vi "Main.vi"(11 "Module Admin":refnum<class "Delacor_lib_QMH_Module Admin.lvclass">) -> ()   [LabVIEW 2024, in "Singleton.lvlib"]
doc: "This template is based off of the Queued Message Handler design pattern and the Queued Message Handler project template that ships with LabVIEW.\n\nThe main difference is that the queue is private to this module and communication between modules is performed via Broadcast and Request events.\n\nRequest events are wrapped in public API methods and are handled in the Event Handling Loop (EHL) of this VI. Any module can register for Broadcast events sent by this module. The EHL generates messages based on user interface actions.\n\nThe Message Handling Loop (MHL) processes messages generated by the EHL, or by other messages. The messages are string values, so new messages can be added easily to the Message Cases case structure in the MHL. Each message cluster can also provide an optional value for Message Data, which is a variant that can be converted to whatever message-specific data is required.\n_____\nBased on DQMH Dev Tools: Project Template 7.1.0.1464."
uses:
  Singleton.lvlib
  <vilib>/Delacor/Delacor QMH/Libraries/Module Admin_class/Delacor_lib_QMH_Module Admin.lvclass
  Module Data--cluster.ctl
  Do Something Argument--cluster.ctl
  <vilib>/Delacor/Delacor QMH/Libraries/Message Queue_class/Delacor_lib_QMH_Message Queue.lvclass/Delacor_lib_QMH_Message Queue.ctl
  Do Something Else Argument--cluster.ctl
  Do Something Else and Wait for Reply Argument--cluster.ctl
  Do Something Else and Wait (Reply Payload)--cluster.ctl
  Stop Argument--cluster.ctl
  <vilib>/Delacor/Delacor QMH/Libraries/Module Admin_class/Delacor_lib_QMH_Module Admin.lvclass/Delacor_lib_QMH_Module Admin.ctl
  New Event Argument--cluster.ctl
  <vilib>/Utility/miscctls.llb/LVPointTypeDef.ctl
  <vilib>/Delacor/Delacor QMH/Libraries/Message Queue_class/Delacor_lib_QMH_Enqueue Message (Single).vi
  <vilib>/Delacor/Delacor QMH/Libraries/Module Admin_class/Delacor_lib_QMH_Get External Launch.vi
  <vilib>/JKI/JKI Simple Localization/Private/RegisterVIJKI_Simple_Localization.vi
  <vilib>/Delacor/Delacor QMH/Libraries/Message Queue_class/Delacor_lib_QMH_Message Queue.lvclass
  <vilib>/JKI/JKI Simple Localization/API/JKI Simple LocalizationJKI_Simple_Localization.lvlib
panel:
  out "error out":errorcluster
  out "X":dbl
  out "Status":string
  in  "Simulate MHL Error":bool
  in  "Simulate EHL Error":bool
  in  "Do Something Else <Replace Me>":bool
  in  "Do Something <Replace Me>":bool
  # "These controls have associated \"Value Changed\" events configured in the Event Structure on the diagram.\n\nReplace them (and reconfigure the Event Structure) with the controls you need for your application. \n\nOther processes communicate with this Module via its Public API (wrappers for its Request Events).\n\nThis Module communicates with other processes via its Broadcast Events.\nAny process that wants to receive these messages can register for this module's Broadcast events."
  # "This template is for the DQMH framework. See the block diagram for more information on how to use this template."
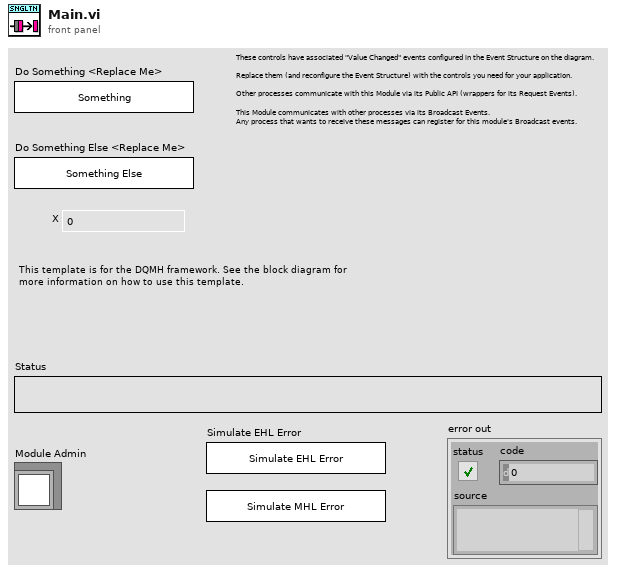
[diagram p1: front panel]
types:
  T1 = typedef "Singleton.lvlib/Request Events--cluster.ctl" = cluster{"Stop Module":refnum<user-event>, "Do Something":refnum<user-event>, "Do Something Else":refnum<user-event>, "Do Something Else and Wait for Reply":refnum<user-event>, "Show Panel":refnum<user-event>, "Hide Panel":refnum<user-event>, "Get Module Execution Status":refnum<user-event>, "Show Diagram":refnum<user-event>, "New Event":refnum<user-event>, "NEW EVENT TO HL":refnum<user-event>}
  T2 = typedef "Singleton.lvlib/Module Data--cluster.ctl" = cluster{"Status":string}
  T3 = typedef "Singleton.lvlib/Do Something Argument--cluster.ctl" = cluster{"Do Something Msg":string}
  T4 = typedef "Singleton.lvlib/Do Something Else Argument--cluster.ctl" = cluster{"Do Something Else Msg":string, "X":dbl}
  T5 = typedef "Singleton.lvlib/Do Something Else and Wait for Reply Argument--cluster.ctl" = cluster{"Do Something Else Msg":string, "X":dbl, "Wait Notifier":refnum<notifier>, "wait for reply":bool}
  T6 = enum32{"invalid lock state", "Not Locked", "Locked (No Password)", "Password-protected"}
  T7 = typedef "Singleton.lvlib/Stop Argument--cluster.ctl" = cluster{"Origin":string, "Exit via Stop Module Req?":bool, "Wait for Module to stop?":bool}
  T8 = typedef "Singleton.lvlib/New Event Argument--cluster.ctl" = cluster{"Numeric":dbl}
  T9 = typedef "LVPointTypeDef.ctl" = cluster{"Horizontal":i16, "Vertical":i16}
  T10 = enum32{"Invalid", "Standard", "Closed", "Hidden", "Minimized", "Maximized"}
  T11 = typedef "Singleton.lvlib/Do Something Else and Wait (Reply Payload)--cluster.ctl" = cluster{"Value":dbl, "error":errorcluster}
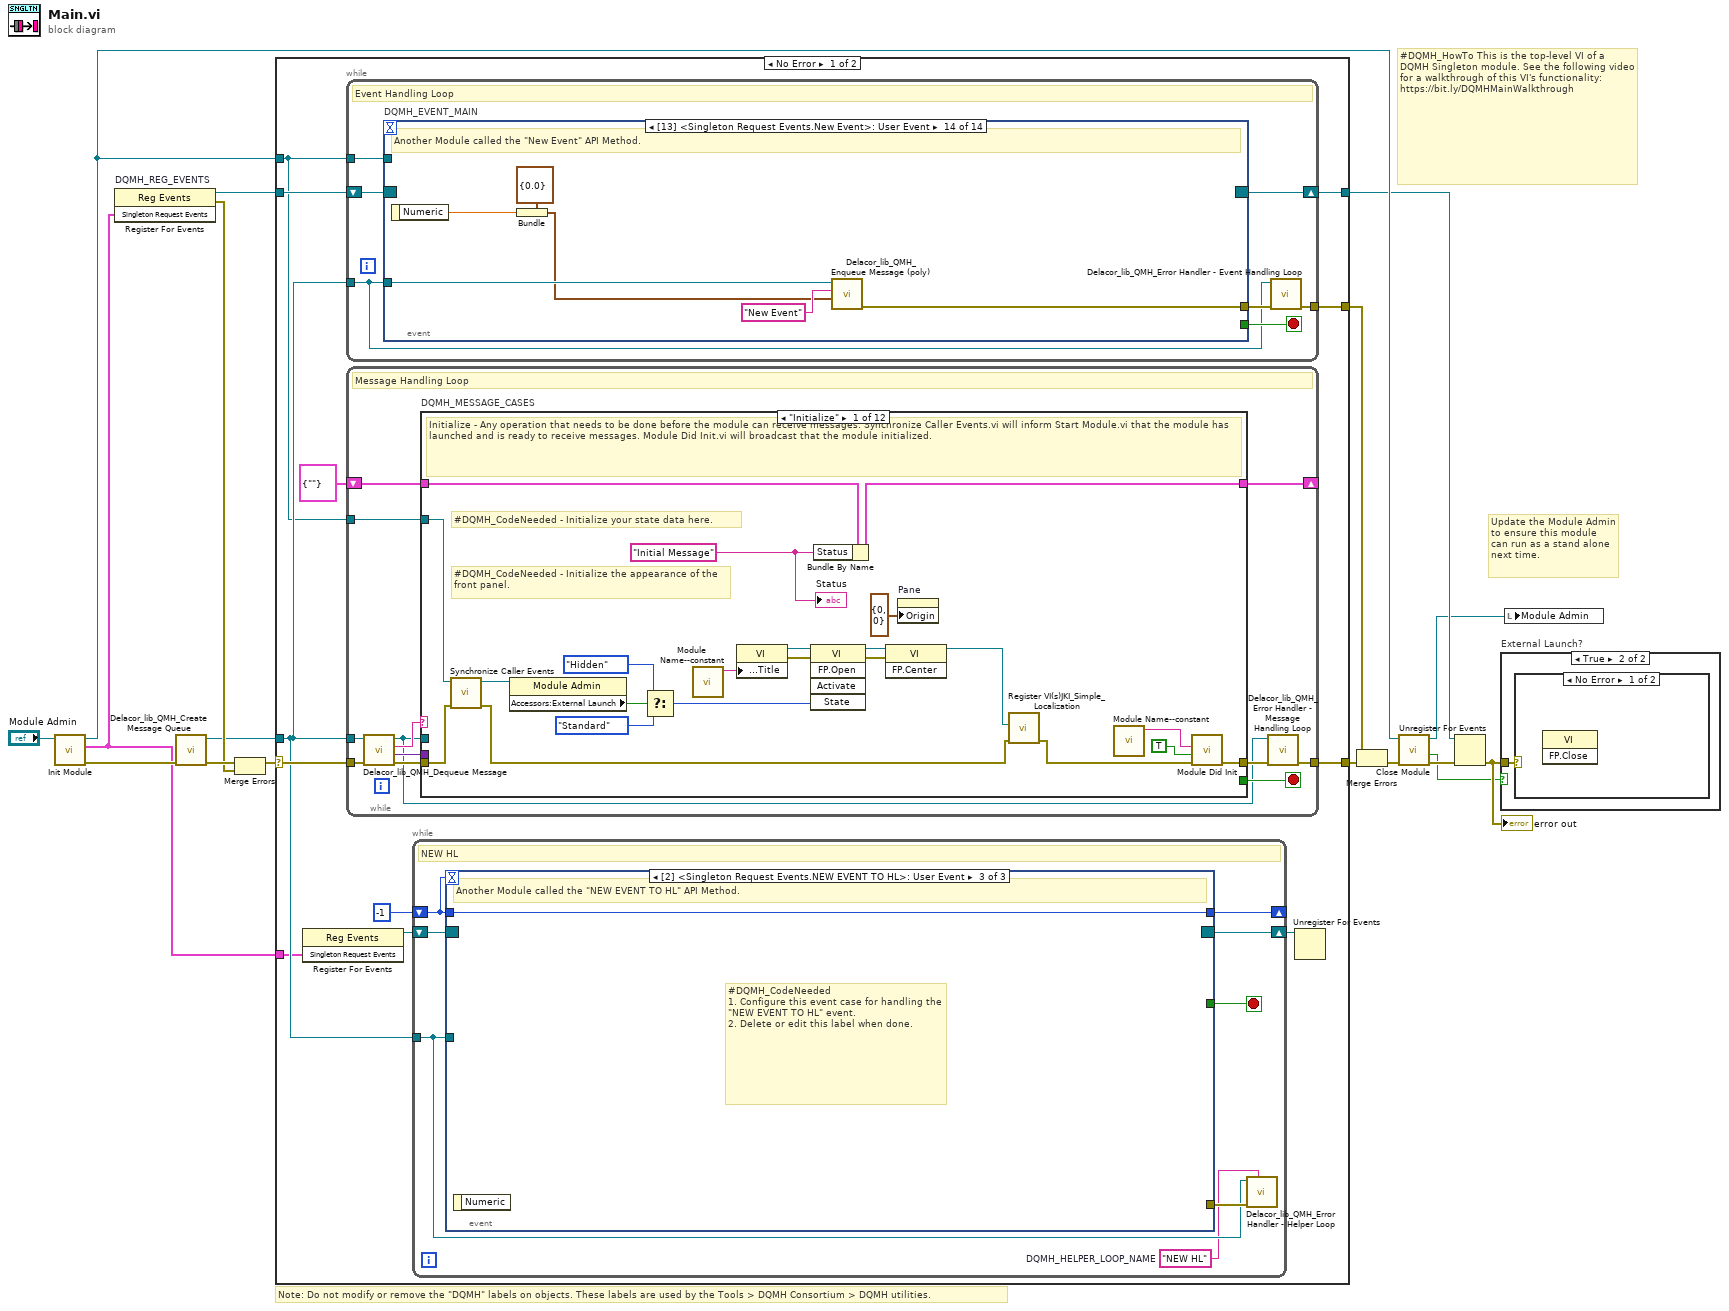
[diagram p0: block diagram]
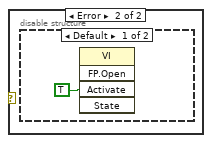
[diagram p3: hidden frame]
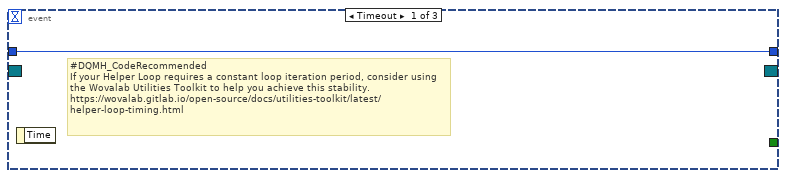
[diagram p5: hidden frame]
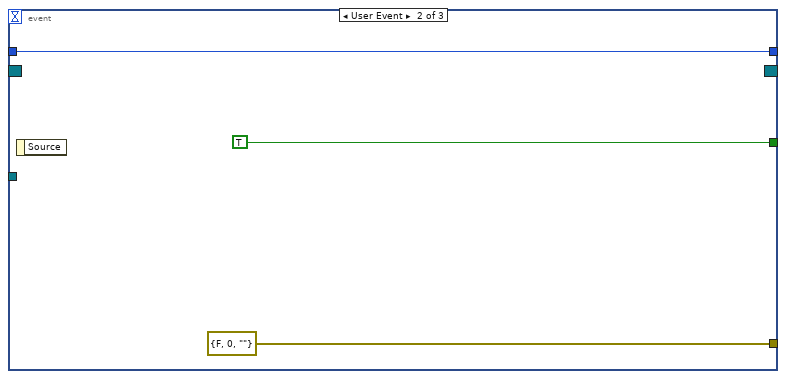
[diagram p6: hidden frame]
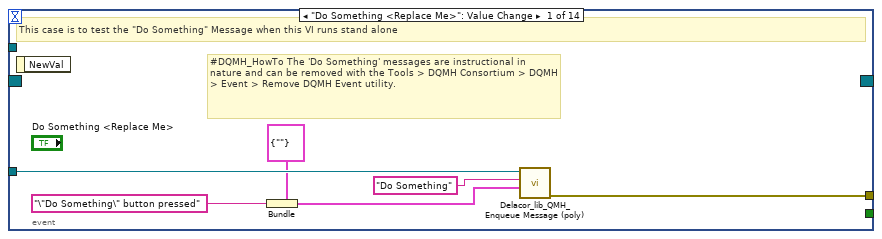
[diagram p7: hidden frame]
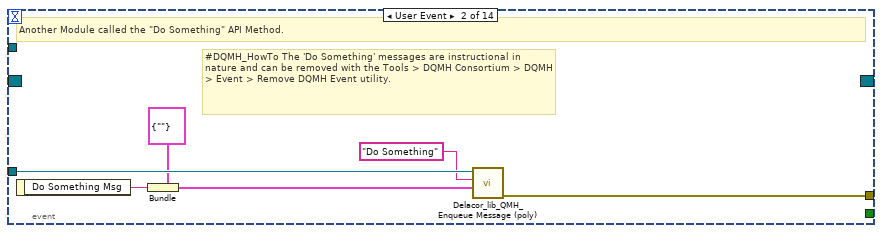
[diagram p8: hidden frame]
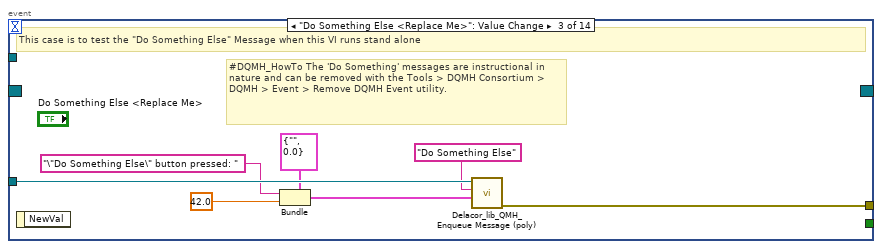
[diagram p9: hidden frame]
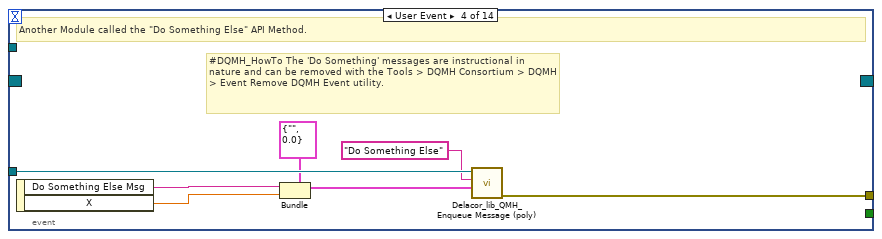
[diagram p10: hidden frame]
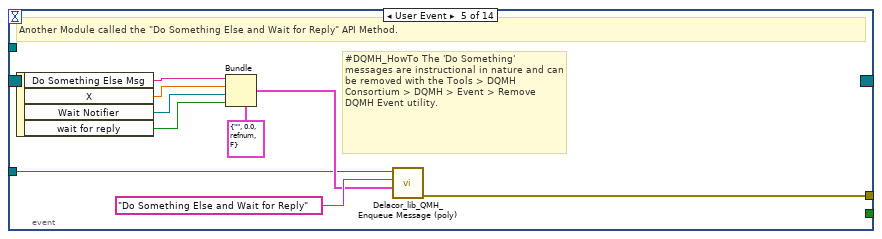
[diagram p11: hidden frame]
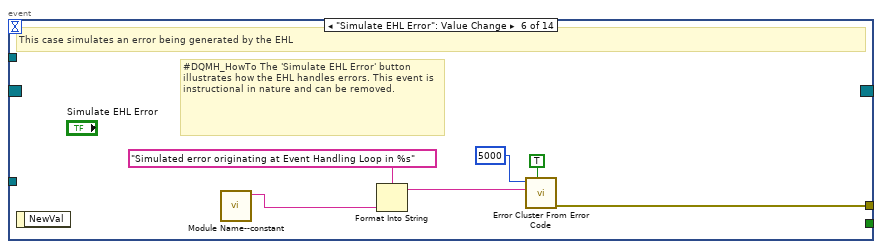
[diagram p12: hidden frame]
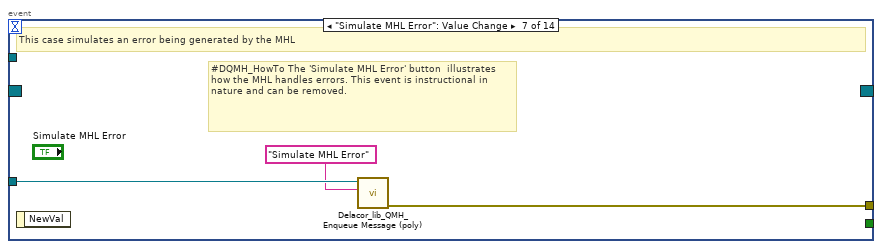
[diagram p13: hidden frame]
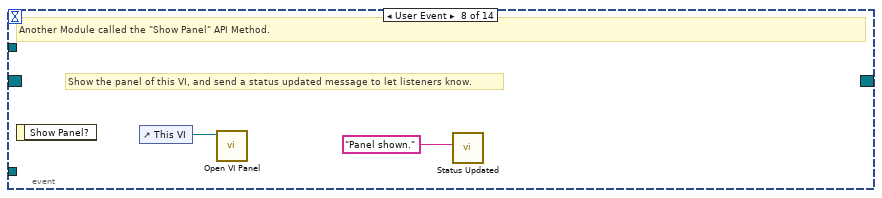
[diagram p14: hidden frame]
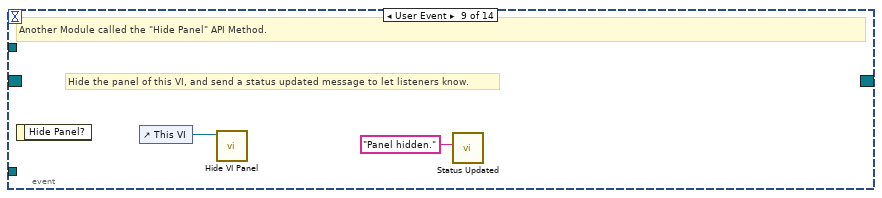
[diagram p15: hidden frame]
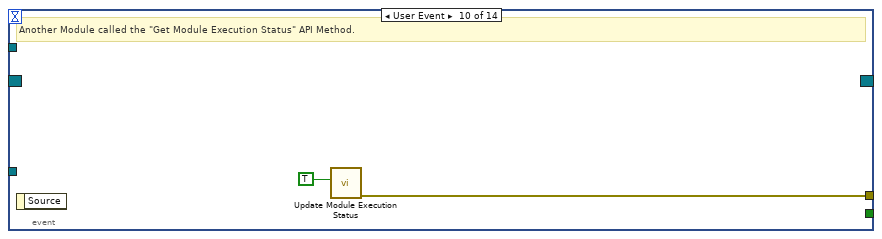
[diagram p16: hidden frame]
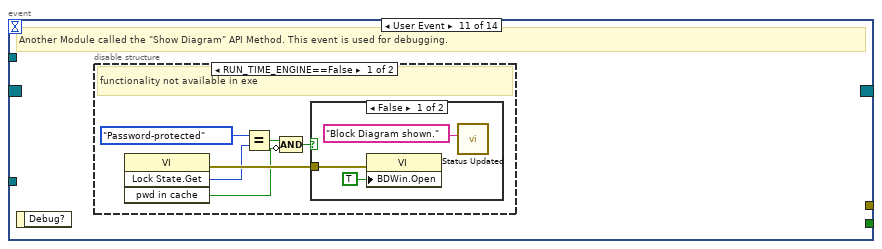
[diagram p17: hidden frame]
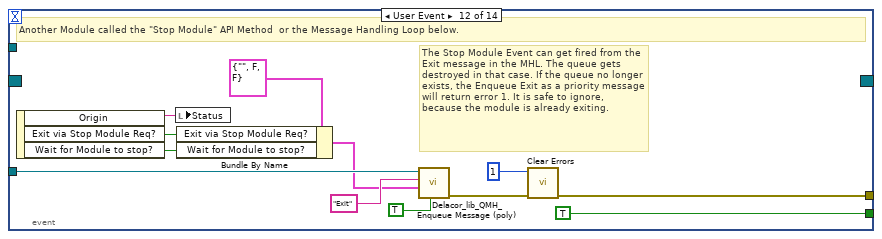
[diagram p20: hidden frame]
diagram:
  # "#DQMH_HowTo This is the top-level VI of a DQMH Singleton module. See the following video for a walkthrough of this VI's functionality: https://bit.ly/DQMHMainWalkthrough"
  # "Note: Do not modify or remove the \"DQMH\" labels on objects. These labels are used by the Tools > DQMH Consortium > DQMH utilities."
  # "Update the Module Admin to ensure this module can run as a stand alone next time."
  n1 = call "Init Module.vi"("Singleton Module Admin in"="Module Admin") -> ("error out"=w16:errorcluster, "Singleton Request Events"=w1:T1, "Singleton Module Admin out"=w8:refnum<class "Delacor_lib_QMH_Module Admin.lvclass">)  [unwired: 8 in]
  n2 = register-events "DQMH_REG_EVENTS"(w1) -> (reference out=w6:refnum<event-registration>, error out=w9:errorcluster)  [unwired: 2 in]
  n3 = call <vilib>:"Delacor_lib_QMH_Create Message Queue.vi"("error in"=w16) -> ("error out"=w11:errorcluster, "Message Queue"=w5:refnum<class "Delacor_lib_QMH_Message Queue.lvclass">)  [unwired: 9 in]
  n4 = Merge Errors(w11, w9) -> (w10:errorcluster)
  n5 = case shown="No Error" w10 {
    selector: w10 -> [w27 w290]
    tunnel: [w29 w289] -> w17
    tunnel: [w26 w288] -> w7
    tunnel: w6 -> [w24 w288]
    tunnel: w5 -> [w23 w283]
    tunnel: [w28 _] -> w14
    tunnel: w8 -> [w22 w284]
    tunnel: w1 -> [w21 _]
    frame No Error {
      n6 = register-events ("DQMH_HELPER_REGFOREVENTS")(w21) -> (reference out=w19:refnum<event-registration>)  [unwired: 2 in, 1 out]
      n7 = while {
        tunnel: w23 -> [w43]
        shift-right: [w46] -> w26
        shift-left: w24 -> [w47]
        tunnel: [w48] -> w28
        tunnel: w22 -> [w44]
        stop <- w45 stop-if-true
        # "Event Handling Loop"
        n8 = event "DQMH_EVENT_MAIN" shown="[13] <Singleton Request Events.New Event>: User Event" {
          selector: w47 -> [_ _ _ _ _ _ _ _ _ _ _ _ _ _]
          dyn-events: [_ _ _ _ _ _ _ _ _ _ _ _ _ _] -> w46
          timeout: _ -> [_ _ _ _ _ _ _ _ _ _ _ _ _ _]
          tunnel: [_ _ _ _ _ _ _ _ _ _ _ TRUE ("Discard?") _ _] -> w45
          tunnel: w43 -> [w54 w60 w67 w74 w77 _ w92 _ _ _ _ w116 w123 w138]
          tunnel: [w55 w61 w68 w75 w84 w90 w93 _ _ w99 _ w119 w125 w133] -> w49
          tunnel: w44 -> [_ _ _ _ _ _ _ _ _ _ _ _ w122 _]
          event "Do Something <Replace Me>": Value Change {
            # "#DQMH_HowTo The 'Do Something' messages are instructional in nature and can be removed with the Tools > DQMH Consortium > DQMH > Event > Remove DQMH Event utility."
            # "This case is to test the \"Do Something\" Message when this VI runs stand alone"
            n9 = event-data() -> ()  [unwired: 1 in, 1 out]
            n10 = Bundle(cluster=T3 {"Do Something Msg"=""} ("Do Something Argument"), "Do Something Msg"="\"Do Something\" button pressed" ("\"Do Something\" button pressed")) -> (w50:T3)
            n11 = call-poly <vilib>:"Delacor_lib_QMH_Enqueue Message (poly).vi"("Message Data"=w50, "Message"="Do Something", "Message Queue in"=w54) -> ("error out"=w55:errorcluster)  [unwired: 7 in, 1 out]
          }
          event User Event {
            # "#DQMH_HowTo The 'Do Something' messages are instructional in nature and can be removed with the Tools > DQMH Consortium > DQMH > Event > Remove DQMH Event utility."
            # "Another Module called the \"Do Something\" API Method."
            n12 = event-data() -> ("Do Something Msg"=w57:string)  [unwired: 1 in]
            n13 = Bundle(cluster=T3 {"Do Something Msg"=""} ("Do Something Argument"), "Do Something Msg"=w57) -> (w56:T3)
            n14 = call-poly <vilib>:"Delacor_lib_QMH_Enqueue Message (poly).vi"("Message Data"=w56, "Message"="Do Something", "Message Queue in"=w60) -> ("error out"=w61:errorcluster)  [unwired: 7 in, 1 out]
          }
          event "Do Something Else <Replace Me>": Value Change {
            # "#DQMH_HowTo The 'Do Something' messages are instructional in nature and can be removed with the Tools > DQMH Consortium > DQMH > Event > Remove DQMH Event utility."
            # "This case is to test the \"Do Something Else\" Message when this VI runs stand alone"
            n15 = event-data() -> ()  [unwired: 1 in, 1 out]
            n16 = Bundle(cluster=T4 {"Do Something Else Msg"="", "X"=0.0} ("Do Something Else Argument"), "Do Something Else Msg"="\"Do Something Else\" button pressed: " ("\"Do Something Else\" button pressed"), "X"=42.0) -> (w64:T4)
            n17 = call-poly <vilib>:"Delacor_lib_QMH_Enqueue Message (poly).vi"("Message Data"=w64, "Message"="Do Something Else", "Message Queue in"=w67) -> ("error out"=w68:errorcluster)  [unwired: 7 in, 1 out]
          }
          event User Event {
            # "#DQMH_HowTo The 'Do Something' messages are instructional in nature and can be removed with the Tools > DQMH Consortium > DQMH > Event Remove DQMH Event utility."
            # "Another Module called the \"Do Something Else\" API Method."
            n18 = event-data() -> ("Do Something Else Msg"=w70:string, "X"=w69:dbl)  [unwired: 1 in]
            n19 = Bundle(cluster=T4 {"Do Something Else Msg"="", "X"=0.0} ("Do Something Else Argument"), "Do Something Else Msg"=w70, "X"=w69) -> (w71:T4)
            n20 = call-poly <vilib>:"Delacor_lib_QMH_Enqueue Message (poly).vi"("Message Data"=w71, "Message"="Do Something Else", "Message Queue in"=w74) -> ("error out"=w75:errorcluster)  [unwired: 7 in, 1 out]
          }
          event User Event {
            # "#DQMH_HowTo The 'Do Something' messages are instructional in nature and can be removed with the Tools > DQMH Consortium > DQMH > Event > Remove DQMH Event utility."
            # "Another Module called the \"Do Something Else and Wait for Reply\" API Method."
            n21 = event-data() -> ("Do Something Else Msg"=w80:string, "X"=w79:dbl, "Wait Notifier"=w78:refnum<notifier>, "wait for reply"=w76:bool)  [unwired: 1 in]
            n22 = Bundle(cluster=T5 {"Do Something Else Msg"="", "X"=0.0, "Wait Notifier"=refnum, "wait for reply"=FALSE} ("Do Something Else and Wait for Reply Argument"), "Do Something Else Msg"=w80, "X"=w79, "Wait Notifier"=w78, "wait for reply"=w76) -> (w81:T5)
            n23 = call-poly <vilib>:"Delacor_lib_QMH_Enqueue Message (poly).vi"("Message Data"=w81, "Message"="Do Something Else and Wait for Reply", "Message Queue in"=w77) -> ("error out"=w84:errorcluster)  [unwired: 7 in, 1 out]
          }
          event "Simulate EHL Error": Value Change {
            # "#DQMH_HowTo The 'Simulate EHL Error' button  illustrates how the EHL handles errors. This event is instructional in nature and can be removed."
            # "This case simulates an error being generated by the EHL"
            n24 = event-data() -> ()  [unwired: 1 in, 1 out]
            n25 = call "Module Name--constant.vi"() -> ("Module Name"=w87:string)  [unwired: 11 in]
            n26 = Format Into String(format string="Simulated error originating at Event Handling Loop in %s", w87) -> (resulting string=w88:string)  [unwired: 2 in, 1 out]
            n27 = call <vilib>:"Error Cluster From Error Code.vi"("show call chain? (False)"=TRUE, "error message (\"\")"=w88, "error code (0)"=5000) -> ("error out"=w90:errorcluster)  [unwired: 6 in]
          }
          event "Simulate MHL Error": Value Change {
            # "#DQMH_HowTo The 'Simulate MHL Error' button  illustrates how the MHL handles errors. This event is instructional in nature and can be removed."
            # "This case simulates an error being generated by the MHL"
            n28 = event-data() -> ()  [unwired: 1 in, 1 out]
            n29 = call-poly <vilib>:"Delacor_lib_QMH_Enqueue Message (poly).vi"("Message"="Simulate MHL Error", "Message Queue in"=w92) -> ("error out"=w93:errorcluster)  [unwired: 8 in, 1 out]
          }
          event User Event {
            # "Show the panel of this VI, and send a status updated message to let listeners know."
            # "Another Module called the \"Show Panel\" API Method."
            n30 = event-data() -> ()  [unwired: 1 in, 1 out]
            n31 = control-ref of="This VI"() -> (w95:refnum<vi>)
            n32 = call "Open VI Panel.vi"("VI"=w95) -> ()  [unwired: 10 in, 1 out]
            n33 = call "Status Updated.vi"("Status"="Panel shown." ("format string")) -> ()  [unwired: 10 in, 1 out]
          }
          event User Event {
            # "Hide the panel of this VI, and send a status updated message to let listeners know."
            # "Another Module called the \"Hide Panel\" API Method."
            n34 = event-data() -> ()  [unwired: 1 in, 1 out]
            n35 = control-ref of="This VI"() -> (w97:refnum<vi>)
            n36 = call "Hide VI Panel.vi"("VI"=w97) -> ()  [unwired: 10 in, 1 out]
            n37 = call "Status Updated.vi"("Status"="Panel hidden." ("format string")) -> ()  [unwired: 10 in, 1 out]
          }
          event User Event {
            # "Another Module called the \"Get Module Execution Status\" API Method."
            n38 = event-data() -> ()  [unwired: 1 in, 1 out]
            n39 = call "Update Module Execution Status.vi"("Running?"=TRUE) -> ("error out"=w99:errorcluster)  [unwired: 10 in]
          }
          event User Event {
            # "Another Module called the \"Show Diagram\" API Method. This event is used for debugging."
            n40 = event-data() -> ()  [unwired: 1 in, 1 out]
            n41 = disable-structure shown="RUN_TIME_ENGINE==False" {
              frame condition #0 (active) {
                # "functionality not available in exe"
                n42 = invoke on="Invoke Node" class="VI" method="Lock State.Get"() -> (error out=w105:errorcluster, "Get Lock State"=w104:T6, "pwd in cache"=w101:bool)  [unwired: 4 in, 1 out]
                n43 = Equal?(x=T6."Password-protected", y=w104) -> (x = y?=w102:bool)
                n44 = Compound Arithmetic op=AND(w102, invert w101) -> (w100:bool)
                n45 = case shown="False" w100 {
                  tunnel: w105 -> [w108 _]
                  frame False {
                    n46 = property on="Property Node" class="VI"(error in=w108, "BDWin.Open"=TRUE ("Block Diagram Window:Open")) -> ()  [unwired: 1 in, 2 out]
                    n47 = call "Status Updated.vi"("Status"="Block Diagram shown." ("format string")) -> ()  [unwired: 10 in, 1 out]
                  }
                  frame True {
                    # "Password-protected VI, and the password is not in the cache. Do not show the diagram."
                  }
                }
              }
              frame condition #1 {
              }
            }
          }
          event User Event {
            # "The Stop Module Event can get fired from the Exit message in the MHL. The queue gets destroyed in that case. If the queue no longer exists, the Enqueue Exit as a priority message will return error 1. It is safe to ignore, because the module is already exiting."
            # "Another Module called the \"Stop Module\" API Method  or the Message Handling Loop below."
            n48 = event-data() -> ("Origin"=w115:string, "Exit via Stop Module Req?"=w111:bool, "Wait for Module to stop?"=w110:bool)  [unwired: 1 in]
            n49 = local write "Status"(w115) -> ()
            n50 = Bundle By Name(cluster=T7 {"Origin"="", "Exit via Stop Module Req?"=FALSE, "Wait for Module to stop?"=FALSE} ("Stop Argument"), "Exit via Stop Module Req?"=w111, "Wait for Module to stop?"=w110) -> (w109:T7)
            n51 = call-poly <vilib>:"Delacor_lib_QMH_Enqueue Message (poly).vi"("Priority Message? (F)"=TRUE, "Message Data"=w109, "Message"="Exit", "Message Queue in"=w116) -> ("error out"=w120:errorcluster)  [unwired: 6 in, 1 out]
            n52 = call <vilib>:"Clear Errors.vi"("error in (no error)"=w120, "specific error code to clear (0: all)"=1) -> ("error out"=w119:errorcluster)  [unwired: 4 in, 1 out]
          }
          event Panel Close? {
            w124 = TRUE  # Discard the event, the MHL is responsible for closing and stopping this VI.
            # "Hide the panel or send the 'Exit' message if the user clicks the 'X' on the module main VI panel."
            n53 = event-data() -> ()  [unwired: 1 in, 1 out]
            n54 = property on="Property Node" class="Module Admin"(reference=w122) -> ("Accessors:External Launch"=w121:bool)  [unwired: 1 in, 2 out]
            n55 = case shown="True" w121 {
              tunnel: w123 -> [_ w131]
              tunnel: [_ w132] -> w125
              frame True {
                # "If externally launched, clicking the 'X' hides the panel, but doesn't close it."
                n56 = control-ref of="This VI"() -> (w128:refnum<vi>)
                n57 = call "Hide VI Panel.vi"("VI"=w128) -> ("error out"=w126:errorcluster)  [unwired: 10 in]
                n58 = call "Status Updated.vi"("error in"=w126, "Status"="Panel hidden." ("format string")) -> ()  [unwired: 9 in, 1 out]
              }
              frame False {
                # "If run as a stand-alone VI, clicking the panel 'X' stops the VI."
                n59 = call-poly <vilib>:"Delacor_lib_QMH_Enqueue Message (poly).vi"("Priority Message? (F)"=TRUE, "Message"="Exit", "Message Queue in"=w131) -> ("error out"=w132:errorcluster)  [unwired: 7 in, 1 out]
              }
            }
            n60 = event-data ("Event Filter Node")("Discard?"=w124) -> ()  [unwired: 1 in, 1 out]
          }
          event User Event {
            # "Another Module called the \"New Event\" API Method."
            n61 = event-data() -> ("Numeric"=w134:dbl)  [unwired: 1 in]
            n62 = Bundle(cluster=T8 {"Numeric"=0.0} ("New Event Argument"), "Numeric"=w134) -> (w135:T8)
            n63 = call-poly <vilib>:"Delacor_lib_QMH_Enqueue Message (poly).vi"("Message Data"=w135, "Message"="New Event", "Message Queue in"=w138) -> ("error out"=w133:errorcluster)  [unwired: 7 in, 1 out]
          }
        }
        n64 = call-dynamic "Delacor_lib_QMH_Error Handler - Event Handling Loop.vi"("error in"=w49, "Message Queue in"=w43) -> ("dup error in"=w48:errorcluster)  [unwired: 8 in, 1 out]
      }
      n65 = while {
        tunnel: w23 -> [w139]
        shift-right: [w147] -> _
        shift-left: T2 {"Status"=""} ("Data Cluster") -> [w148]
        tunnel: w27 -> [w150]
        tunnel: [w142] -> w29
        tunnel: w22 -> [w143]
        stop <- w146 stop-if-true
        # "Message Handling Loop"
        n66 = call-dynamic "Delacor_lib_QMH_Dequeue Message.vi"("error in"=w150, "Message Queue in"=w139) -> ("error out"=w149:errorcluster, "Message Data"=w144:variant, "Message"=w145:string, "Message Queue out"=w140:refnum<class "Delacor_lib_QMH_Message Queue.lvclass">)  [unwired: 6 in]
        n67 = case "DQMH_MESSAGE_CASES" shown="\"Initialize\"" w145 {
          selector: w145 -> [_ _ _ _ _ _ _ _ _ _ _ w278]
          tunnel: w140 -> [_ _ _ _ _ _ _ _ _ w244 w266 _]
          tunnel: w149 -> [w170 w174 w182 w191 w210 w226 w229 w231 w240 w251 w272 w281]
          tunnel: [w169 w174 w180 w190 w209 w224 w228 w231 w239 w247 w267 w282] -> w141
          tunnel: w148 -> [w160 w173 w179 w189 w206 w225 w227 w230 w237 w246 w265 w279]
          tunnel: [w159 w173 w179 w189 w206 w225 w227 w230 w237 w246 w265 w279] -> w147
          tunnel: [_ _ _ _ _ _ _ _ _ _ w264 _] -> w146
          tunnel: w144 -> [_ _ w178 w186 w203 w223 _ _ _ w245 w263 _]
          tunnel: w143 -> [w161 _ _ _ _ _ _ _ _ w243 w258 _]
          frame "Initialize" {
            w155 = "Initial Message" ("Initial Message")
            # "#DQMH_CodeNeeded - Initialize the appearance of the front panel."
            # "#DQMH_CodeNeeded - Initialize your state data here."
            # "Initialize - Any operation that needs to be done before the module can receive messages. Synchronize Caller Events.vi will inform Start Module.vi that the module has launched and is ready to receive messages. Module Did Init.vi will broadcast that the module initialized."
            n68 = call "Synchronize Caller Events.vi"("error in"=w170, "Singleton Module Admin in"=w161) -> ("error out"=w153:errorcluster, "Singleton Module Admin out"=w156:refnum<class "Delacor_lib_QMH_Module Admin.lvclass">)  [unwired: 8 in]
            n69 = property on="Property Node" class="Module Admin"(reference=w156) -> ("Accessors:External Launch"=w165:bool)  [unwired: 1 in, 2 out]
            n70 = Select(t=T10."Hidden" ("State"), s=w165, f=T10."Standard" ("State")) -> (s? t:f=w162:T10)
            n71 = call "Module Name--constant.vi"() -> ("Module Name"=w168:string)  [unwired: 11 in]
            n72 = property on="Property Node" class="VI"("Front Panel.Title"=w168) -> (reference out=w167:refnum<vi>, error out=w172:errorcluster)  [unwired: 2 in]
            n73 = invoke on="Invoke Node" class="VI" method="FP.Open"(reference=w167, error in=w172, "State"=w162) -> (reference out=w166:refnum<vi>, error out=w171:errorcluster)  [unwired: 2 in, 3 out]
            n74 = Bundle By Name(cluster=w160, "Status"=w155) -> (w159:T2)
            n75 = invoke on="Invoke Node" class="VI" method="FP.Center"(reference=w166, error in=w171) -> (reference out=w151:refnum<vi>)  [unwired: 1 in, 2 out]
            n76 = property on="Pane" class="Pane"("Origin"=T9 {"Horizontal"=0, "Vertical"=0}) -> ()  [unwired: 2 in, 2 out]
            n77 = call-poly <vilib>:"Register VI(s)JKI_Simple_Localization.vi"("error in"=w153, "VI Ref"=w151) -> ("error out"=w152:errorcluster)  [unwired: 8 in, 1 out]
            n78 = call "Module Name--constant.vi"() -> ("Module Name"=w157:string)  [unwired: 11 in]
            n79 = call "Module Did Init.vi"("error in"=w152, "Initialized?"=TRUE, "Origin"=w157) -> ("error out"=w169:errorcluster)  [unwired: 8 in]
            "Status" <- w155
          }
          frame "---Module Specific---" {
            # "Separator -- The following cases handle messages specific to this Module."
          }
          frame "Do Something" {
            # "#DQMH_HowTo The 'Do Something' messages are instructional in nature and can be removed with the Tools > DQMH Consortium > DQMH > Event > Remove DQMH Event utility."
            # "Do Something - Replace this message with functionality for your own application. Note that this message also fires the \"Did Something\" broadcast event."
            n80 = Variant To Data(error in=w182, type=T3 {"Do Something Msg"=""} ("Do Something Argument"), Variant=w178) -> (data=w177:T3, error out=w181:errorcluster)
            n81 = Unbundle By Name(w177) -> ("Do Something Msg"=w175:string)
            n82 = call "Did Something.vi"("error in"=w181, "Did Something Msg"=w175) -> ("error out"=w180:errorcluster)  [unwired: 9 in]
            n83 = local write "Status"(w175) -> ()
            n84 = call "Status Updated.vi"("Status"=w175) -> ()  [unwired: 10 in, 1 out]
          }
          frame "Do Something Else" {
            # "#DQMH_HowTo The 'Do Something' messages are instructional in nature and can be removed with the Tools > DQMH Consortium > DQMH > Event > Remove DQMH Event utility."
            # "Do Something Else - Replace this message with functionality for your own application."
            n85 = Variant To Data(error in=w191, type=T4 {"Do Something Else Msg"="", "X"=0.0} ("Do Something Else Argument"), Variant=w186) -> (data=w187:T4, error out=w190:errorcluster)
            n86 = Unbundle By Name(w187) -> ("Do Something Else Msg"=w185:string, "X"=w184:dbl)
            "X" <- w184
            n87 = Format Into String(initial string=w185, w184) -> (resulting string=w183:string)  [unwired: 2 in, 1 out]
            n88 = local write "Status"(w183) -> ()
            n89 = call "Status Updated.vi"("Status"=w183) -> ()  [unwired: 10 in, 1 out]
          }
          frame "Do Something Else and Wait for Reply" {
            w198 = "X(%.2f)+Offset(%.2f)=%.2f"  # status message format string
            # "#DQMH_HowTo The 'Do Something' messages are instructional in nature and can be removed."
            # "Send back X with a random offset"
            # "Do Something Else and Wait for Reply - Replace this message with functionality for your own application. Note that this message must fire a notifier to let callers know it has finished execution, and it returns an error if the 'Value' is negative."
            n90 = Variant To Data(error in=w210, type=T5 {"Do Something Else Msg"="", "X"=0.0, "Wait Notifier"=refnum, "wait for reply"=FALSE} ("Do Something Else and Wait for Reply Argument"), Variant=w203) -> (data=w204:T5, error out=w208:errorcluster)
            n91 = Unbundle By Name(w204) -> ("Wait Notifier"=w192:refnum<notifier>, "Do Something Else Msg"=w202:string, "X"=w199:dbl, "wait for reply"=w195:bool)
            n92 = Random Number (0-1)() -> (number: 0 to 1=w200:dbl)
            n93 = Add(x=w200, y=w199) -> (x+y=w194:dbl)
            n94 = Less Than 0?(x=w194) -> (x < 0?=w197:bool)
            n95 = local write "X"(w199) -> ()
            n96 = case shown="True" w197 {
              tunnel: [_ w220] -> w207
              frame False {
              }
              frame True {
                n97 = call <vilib>:"Error Cluster From Error Code.vi"("show call chain? (False)"=TRUE, "error message (\"\")"="The 'Something Else and Wait for Reply' message generated a negative number, which is considered an error condition.", "error code (0)"=5000) -> ("error out"=w220:errorcluster)  [unwired: 6 in]
              }
            }
            n98 = Format Into String(format string=w198, initial string=w202, w199, w200, w194) -> (resulting string=w196:string)  [unwired: 1 in, 1 out]
            n99 = Bundle By Name(cluster=T11 {"Value"=0.0, "error"={"status"=FALSE, "code"=0, "source"=""}} ("notification"), "error"=w207, "Value"=w194) -> (w193:T11)
            n100 = local write "Status"(w196) -> ()
            n101 = call "Status Updated.vi"("Status"=w196) -> ()  [unwired: 10 in, 1 out]
            n102 = case shown="True" w195 {
              tunnel: w193 -> [_ w213]
              tunnel: w192 -> [_ w212]
              frame False {
              }
              frame True {
                # "Simulate an operation that requires a wait."
                n103 = flat-sequence {
                  tunnel: w213 -> [w216]
                  tunnel: w212 -> [w215]
                  tunnel: w211 -> [_]
                  frame #0 {
                    n104 = Send Notification(notification=w216, notifier=w215) -> ()  [unwired: 1 in, 2 out]
                  }
                }
                n105 = Wait (ms)(milliseconds to wait=u32 1000) -> (millisecond timer value=w211:u32)
              }
            }
            n106 = Merge Errors(w208, w207) -> (w209:errorcluster)
          }
          frame "New Event" {
            # "#DQMH_CodeNeeded\n1. Configure this Message Case for handling the \"New Event\" message.\n2. Delete or edit this label when done."
            # "New Event Documentation"
            n107 = Variant To Data(error in=w226, type=T8 {"Numeric"=0.0} ("New Event Argument"), Variant=w223) -> (data=w221:T8, error out=w224:errorcluster)
            n108 = Unbundle By Name(w221) -> ()  [unwired: 1 out]
          }
          frame "---Copy This Frame---" {
            # "Duplicate this frame when creating new messages.  Change this comment in the duplicated frame to describe this message."
            n109 = Merge Errors(w229) -> (w228:errorcluster)
          }
          frame "---Exit and Error Handling---" {
            # "Separator - The following cases handle errors and exit messages."
          }
          frame "Simulate MHL Error" {
            # "#DQMH_HowTo The 'Simulate MHL Error' button  illustrates how the MHL handles errors. This event is instructional in nature and can be removed."
            # "Simulate an error occurring at the MHL"
            n110 = call "Module Name--constant.vi"() -> ("Module Name"=w233:string)  [unwired: 11 in]
            n111 = Format Into String(format string="Simulated error originating at Message Handling Loop in %s", w233) -> (resulting string=w234:string)  [unwired: 2 in, 1 out]
            n112 = call <vilib>:"Error Cluster From Error Code.vi"("show call chain? (False)"=TRUE, "error message (\"\")"=w234, "error code (0)"=5001) -> ("error out"=w238:errorcluster)  [unwired: 6 in]
            n113 = Merge Errors(w240, w238) -> (w239:errorcluster)
          }
          frame "Error" {
            # "#DQMH_CodeRecommended - If the module is running in standalone mode (External Launch = FALSE), this code will pop up an error dialog and call the 'Exit' message if an error occurs. Add more fine-grained error management here."
            # "Error - Check the error message data and respond accordingly. This message is sent by the \"Error Handler\" VIs at the end of each loop in this application."
            n114 = property on="Property Node" class="Module Admin"(reference=w243) -> ("Accessors:External Launch"=w242:bool)  [unwired: 1 in, 2 out]
            n115 = Variant To Data(error in=w251, type=errorcluster {"status"=FALSE, "code"=0, "source"=""} ("error constant"), Variant=w245) -> (data=w241:errorcluster, error out=w249:errorcluster)
            n116 = local write "error out"(w241) -> ()
            n117 = call "Error Reported.vi"("Error"=w241) -> ()  [unwired: 10 in, 1 out]
            n118 = case shown="False" w242 {
              tunnel: [w256 _] -> w248
              tunnel: w244 -> [w254 _]
              tunnel: w241 -> [w255 _]
              frame False {
                n119 = disable-structure shown="Default" {
                  disable-tunnel: w255 -> [w257 _]
                  frame condition #0 (active) {
                    # "If the module is running standalone, then pop up an error dialog and call the \"Exit\" message."
                    n120 = call <vilib>:"Simple Error Handler.vi"("error in (no error)"=w257) -> ()  [unwired: 4 in, 5 out]
                  }
                  frame condition #1 {
                    # "To prevent the Simple Error Handler VI from being loaded (e.g. when deploying to a Real-Time target), add the Conditional Disable Symbol \"DQMH_Disable_SEH\" to your project and set it to TRUE."
                  }
                }
                n121 = call-poly <vilib>:"Delacor_lib_QMH_Enqueue Message (poly).vi"("Priority Message? (F)"=TRUE, "Message"="Exit", "Message Queue in"=w254) -> ("error out"=w256:errorcluster)  [unwired: 7 in, 1 out]
              }
              frame True {
                # "If the module was launched externally, calling the Error Reported broadcast VI is the only action performed by the \"Error\" message. The module's caller can then process the error appropriately."
              }
            }
            n122 = Merge Errors(w249, w248) -> (w247:errorcluster)
          }
          frame "Exit" {
            w262 = 91  # 91: not all Exit messages will have an argument
            w264 = TRUE  # Stop the VI
            # "Release the message queue reference"
            # "#DQMH_CodeNeeded - Add any required cleanup code here."
            # "Exit - Exit the application."
            n123 = Variant To Data(error in=w272, type=T7 {"Origin"="", "Exit via Stop Module Req?"=FALSE, "Wait for Module to stop?"=FALSE} ("Stop Argument"), Variant=w263) -> (data=w260:T7, error out=w269:errorcluster)
            n124 = call <vilib>:"Clear Errors.vi"("error in (no error)"=w269, "specific error code to clear (0: all)"=w262) -> ("error out"=w271:errorcluster)  [unwired: 4 in, 1 out]
            n125 = control-ref of="This VI"() -> (w259:refnum<vi>)
            n126 = call-dynamic "Delacor_lib_QMH_Release Message Queue.vi"("error in"=w271, "Message Queue"=w266) -> ("error out"=w270:errorcluster)  [unwired: 9 in]
            n127 = call "Handle Exit.vi"("Stop Argument"=w260, "Admin in"=w258, "VI reference"=w259) -> ("error out"=w268:errorcluster)  [unwired: 7 in, 1 out]
            n128 = Merge Errors(w270, w268) -> (w267:errorcluster)
            n129 = call "Error Reported.vi"("Error"=w267) -> ()  [unwired: 10 in, 1 out]
          }
          frame Default {
            # "'Default' case only runs if there is a message that isn't defined in any of the other cases.  Output a programming error."
            n130 = call "Module Name--constant.vi"() -> ("Module Name"=w277:string)  [unwired: 11 in]
            n131 = Format Into String(format string="The invalid message string \"%s\" was received in the Message Handling Loop for module \"%s\".", w278, w277) -> (resulting string=w273:string)  [unwired: 2 in, 1 out]
            n132 = call <vilib>:"Error Cluster From Error Code.vi"("show call chain? (False)"=TRUE, "error message (\"\")"=w273, "error code (0)"=1) -> ("error out"=w280:errorcluster)  [unwired: 6 in]
            n133 = Merge Errors(w281, w280) -> (w282:errorcluster)
          }
        }
        n134 = call-dynamic "Delacor_lib_QMH_Error Handler - Message Handling Loop.vi"("error in"=w141, "Message Queue in"=w140) -> ("dup error in"=w142:errorcluster)  [unwired: 8 in, 1 out]
      }
      n135 = while "DQMH_HELPER_LOOP" {
        shift-right: [w37] -> _
        shift-left: -1 -> [w36]
        shift-right: [w34] -> w20
        shift-left: w19 -> [w35]
        tunnel: w23 -> [w31]
        stop <- w33 stop-if-true
        w30 = "NEW HL"  # DQMH_HELPER_LOOP_NAME
        # "NEW HL"
        n136 = event "DQMH_HELPER_EVENT_STRUCTURE" shown="[2] <Singleton Request Events.NEW EVENT TO HL>: User Event" {
          selector: w35 -> [_ _ _]
          dyn-events: [_ _ _] -> w34
          timeout: w36 -> [_ _ _]
          tunnel: w36 -> [w38 w41 w42]
          tunnel: [w38 w41 w42] -> w37
          tunnel: [_ TRUE _] -> w33
          tunnel: [_ errorcluster {"status"=FALSE, "code"=0, "source"=""} ("error constant") _] -> w32
          tunnel: w31 -> [_ _ _]
          event Timeout {
            # "#DQMH_CodeRecommended\nIf your Helper Loop requires a constant loop iteration period, consider using the Wovalab Utilities Toolkit to help you achieve this stability.\nhttps://wovalab.gitlab.io/open-source/docs/utilities-toolkit/latest/helper-loop-timing.html"
            n137 = event-data() -> ()  [unwired: 1 in, 1 out]
          }
          event User Event {
            n138 = event-data() -> ()  [unwired: 1 in, 1 out]
          }
          event User Event {
            # "#DQMH_CodeNeeded\n1. Configure this event case for handling the \"NEW EVENT TO HL\" event.\n2. Delete or edit this label when done."
            # "Another Module called the \"NEW EVENT TO HL\" API Method."
            n139 = event-data() -> ()  [unwired: 1 in, 1 out]
          }
        }
        n140 = call-dynamic "Delacor_lib_QMH_Error Handler - Helper Loop.vi"("Error Debug"=w30, "error in"=w32, "Message Queue in"=w31) -> ()  [unwired: 7 in, 2 out]
      }
      n141 = Unregister For Events(event registration refnum=w20) -> ()  [unwired: 1 in, 1 out]
    }
    frame Error {
      # "Synchronize Caller Events.vi will inform Start Module.vi that the module has launched and will let the code calling Start Module.vi register for broadcasts and would permit the caller receive the broadcast that an error occurred at launch time."
      n142 = call-dynamic "Delacor_lib_QMH_Release Message Queue.vi"("error in"=w290, "Message Queue"=w283) -> ("error out"=w289:errorcluster)  [unwired: 9 in]
      n143 = call "Synchronize Caller Events.vi"("Singleton Module Admin in"=w284) -> ("error out"=w291:errorcluster)  [unwired: 9 in, 1 out]
      n144 = call "Module Name--constant.vi"() -> ("Module Name"=w287:string)  [unwired: 11 in]
      n145 = Format Into String(format string="An error occurred during initialization. %s is no longer running.", w287) -> (resulting string=w285:string)  [unwired: 2 in, 1 out]
      n146 = Merge Errors(w289, w291) -> (w292:errorcluster)
      n147 = call "Error Reported.vi"("Additional Information"=w285, "Error"=w292) -> ()  [unwired: 9 in, 1 out]
    }
  }
  n148 = Merge Errors(w14, w17) -> (w13:errorcluster)
  n149 = call "Close Module.vi"("error in"=w13, "Module Admin in"=w8) -> ("error out"=w15:errorcluster, "External Launch"=w2:bool, "Module Admin out"=w3:refnum<class "Delacor_lib_QMH_Module Admin.lvclass">)  [unwired: 7 in]
  n150 = Unregister For Events(event registration refnum=w7, error in=w15) -> (error out=w12:errorcluster)
  "error out" <- w12
  n151 = case "External Launch?" shown="True" w2 {
    tunnel: w12 -> [_ w293]
    frame False {
    }
    frame True {
      n152 = case shown="No Error" w293 {
        frame No Error {
          n153 = invoke on="Invoke Node" class="VI" method="FP.Close"() -> ()  [unwired: 3 in, 3 out]
        }
        frame Error {
          n154 = disable-structure shown="Default" {
            frame condition #0 (active) {
              n155 = invoke class="VI" method="FP.Open"("Activate"=TRUE ("Activate?")) -> ()  [unwired: 4 in, 5 out]
            }
            frame condition #1 {
              # "Don't show panel on error if running inside a built EXE."
            }
          }
        }
      }
    }
  }
  n156 = local write "Module Admin"(w3) -> ()
